vi "usb set Port Disable.vi"(7 "dll path in":path, 8 "error in (no error)":errorcluster, 9 "channel":u8, 10 "result":cluster{"value":i32, "error":i32}, 11 "id":u32) -> (0 "error out":errorcluster, 2 "result out":cluster{"value":i32, "error":i32}, 3 "id out":u32)   [LabVIEW 2025]
doc: "aLIBEXPORT void __stdcall usb_setPortDisable ( unsigned int* id, struct Result* result , const unsigned char channel ) ;"
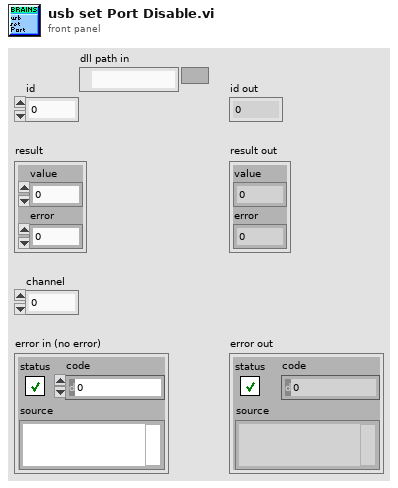
[diagram p1: front panel]
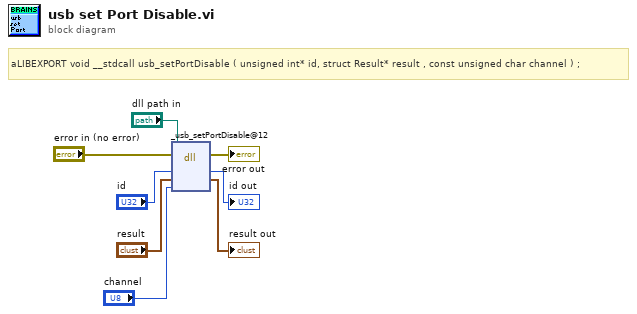
[diagram p0: block diagram]
diagram:
  # "aLIBEXPORT void __stdcall usb_setPortDisable ( unsigned int* id, struct Result* result , const unsigned char channel ) ;"
  n1 = dll-call lib="?" fn="_usb_setPortDisable@12"(path in="dll path in", error in="error in (no error)", "id"="id", "result"="result", "channel"="channel") -> (error out=→"error out":errorcluster, "id"=→"id out":u32, "result"=→"result out":cluster{"value":i32, "error":i32})  [unwired: 3 in, 1 out]
